vi "visitMonitor_RegArray.vi"(0 "HGF_Event":refnum<class "HGF_Event.lvclass">, 5 "error in (no error)":errorcluster) -> (15 "timed out?":bool, 16 "Registration Array":T1(array[cluster]), 19 "error out":errorcluster)   [LabVIEW 2009, in "MoAgSy.lvlib" / "MoAgSy_Host.lvclass"]
uses:
  MoAgSy_Host.lvclass
  HGF_BaseClasses/HGF_Event/HGF_Event.lvclass
  HGF_BaseClasses/HGF_NetworkVisitor/HGF_NetworkVisitor.lvclass
  HGF_BaseClasses/HGF_TriggeredEvent/HGF_TriggeredEvent.lvclass
  HGF_SV/Visitors/HGF_SVMonitorVisitor_getReg/HGF_SVMonitorVisitor_getReg.lvclass
  HGF_BaseClasses/HGF_Notifier/HGF_Notifier.lvclass
  HGF_SV/HGF_SVFactory/HGF_SVFactory.lvclass
  HGF_BaseClasses/HGF_Visitor/HGF_Visitor.lvclass
  HGF_BaseClasses/HGF_Factory/HGF_Factory.lvclass
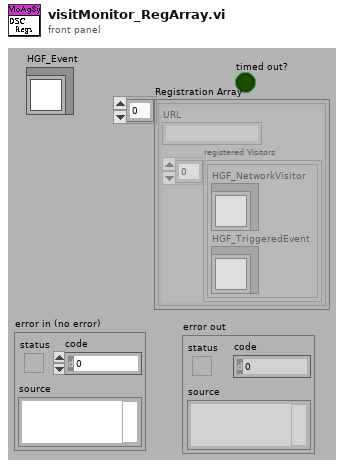
[diagram p1: front panel]
types:
  T1 = cluster{"URL":string, "registered Visitors":cluster{"HGF_NetworkVisitor":refnum<class "HGF_NetworkVisitor.lvclass">, "HGF_TriggeredEvent":refnum<class "HGF_TriggeredEvent.lvclass">}[]}[]
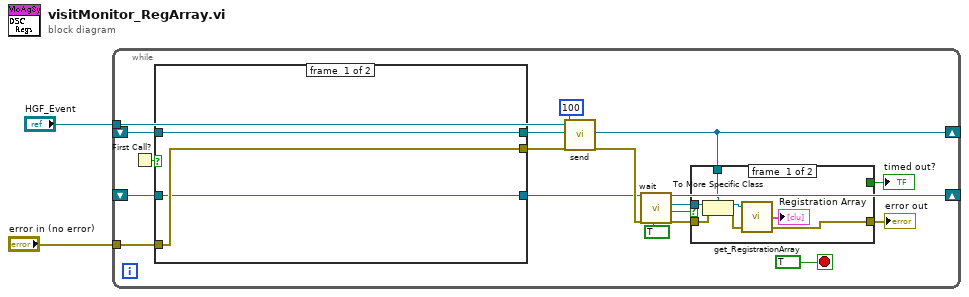
[diagram p0: block diagram]
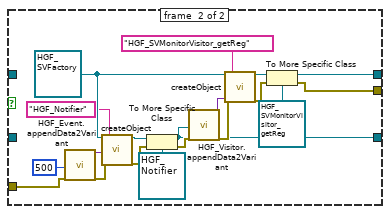
[diagram p3: hidden frame]
diagram:
  n1 = while {
    tunnel: "HGF_Event" -> [w15]
    tunnel: "error in (no error)" -> [w17]
    shift-right: [w7] -> _
    shift-left: _ -> [w6]
    shift-right: [w5] -> _
    shift-left: _ -> [w4]
    stop <- TRUE stop-if-true
    n2 = First Call?() -> (First Call?: T/F=w19:bool)
    n3 = case shown="True" w19 {
      tunnel: [w30 w36] -> w5
      tunnel: [w31 w35] -> w13
      tunnel: w17 -> [w32 w34]
      tunnel: [w32 w33] -> w16
      tunnel: w6 -> [w31 _]
      tunnel: w4 -> [w30 _]
      frame #0 {
      }
      frame #1 {
        w49 = refnum<class "HGF_SVFactory.lvclass"> refnum ("HGF_SV.lvlib:HGF_SVFactory.lvclass")
        n4 = call "HGF_Event.appendData2Variant.vi"("timeout in ms (-1)"=500, "error in (no error)"=w34) -> ("dup initData"=w47:variant, "error out"=w41:errorcluster)  [unwired: 16 in]
        n5 = call "createObject.vi"("HGF_Factory"=w49, "initializationData"=w47, "error in (no error)"=w41, "className"="HGF_Notifier") -> ("HGF_Object"=w45:refnum<class "HGF_Factory.lvclass">, "error out"=w40:errorcluster)  [unwired: 13 in, 1 out]
        n6 = To More Specific Class(target class=refnum<class "HGF_Notifier.lvclass"> refnum ("HGF_BaseClasses.lvlib:HGF_Notifier.lvclass"), reference=w45, error in=w40) -> (specific class reference=w35:refnum<class "HGF_Notifier.lvclass">, error out=w39:errorcluster)
        n7 = call "HGF_Visitor.appendData2Variant.vi"("destination"=w35, "error in (no error)"=w39) -> ("dup initData"=w51:variant, "error out"=w38:errorcluster)  [unwired: 16 in]
        n8 = call "createObject.vi"("HGF_Factory"=w49, "initializationData"=w51, "error in (no error)"=w38, "className"="HGF_SVMonitorVisitor_getReg") -> ("HGF_Object"=w43:refnum<class "HGF_Factory.lvclass">, "error out"=w37:errorcluster)  [unwired: 13 in, 1 out]
        n9 = To More Specific Class(target class=refnum<class "HGF_SVMonitorVisitor_getReg.lvclass"> refnum ("HGF_SV.lvlib:HGF_SVMonitorVisitor_getReg.lvclass"), reference=w43, error in=w37) -> (specific class reference=w36:refnum<class "HGF_SVMonitorVisitor_getReg.lvclass">, error out=w33:errorcluster)
      }
    }
    n10 = call-dynamic "send.vi"("HGF_Event"=w15, "Object"=w5, "timeout in ms (-1)"=100, "error in (no error)"=w16) -> ("error out"=w14:errorcluster)  [unwired: 13 in, 2 out]
    n11 = call-dynamic "wait.vi"("HGF_Notifier"=w13, "error in (no error)"=w14, "ignore previous (F)"=TRUE) -> ("dup HGF_Notifier"=w7:refnum<class "HGF_Notifier.lvclass">, "Object"=w12:refnum<class>, "timed out"=w11:bool, "error out"=w10:errorcluster)  [unwired: 13 in]
    n12 = case shown="False" w11 {
      selector: w11 -> [_ w28]
      tunnel: w5 -> [w25 _]
      tunnel: w12 -> [w24 _]
      tunnel: w10 -> [w23 w29]
      tunnel: [w22 w29] -> w9
      tunnel: [_ w28] -> w8
      frame #0 {
        n13 = To More Specific Class(target class=w25, reference=w24, error in=w23) -> (specific class reference=w26:refnum<class "HGF_SVMonitorVisitor_getReg.lvclass">, error out=w27:errorcluster)
        n14 = call "get_RegistrationArray.vi"("error in (no error)"=w27, "HGF_SVMonitorVisitor_getReg in"=w26) -> ("error out"=w22:errorcluster, "Registration Array"=→"Registration Array":T1)  [unwired: 1 in, 1 out]
      }
      frame #1 {
      }
    }
    "error out" <- w9
    "timed out?" <- w8
  }
